vi "Build Action Array.vi"(10 "directions":T2[](array[typedef]), 11 "Action":T1=enum."Move") -> (3 "actions":cluster{"Action":T1, "Direction":T2}[](array[cluster]))   [LabVIEW 2015, in "DS Square.lvlib"]
uses:
  DS Square.lvlib
  Type Defs/Direction Enum.ctl
  Type Defs/SB Type Defs.lvlib
  Type Defs/Action Enum.ctl
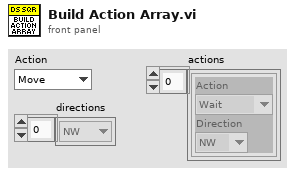
[diagram p1: front panel]
types:
  T1 = typedef "SB Type Defs.lvlib/Action Enum.ctl" = enum16{"Wait", "Move", "Attack", "Replicate"}
  T2 = typedef "SB Type Defs.lvlib/Direction Enum.ctl" = enum16{"NW", "N", "NE", "E", "SE", "S", "SW", "W"}
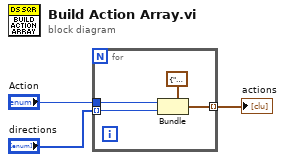
[diagram p0: block diagram]
diagram:
  n1 = for {
    tunnel: "directions" -> [w7] mode=indexing
    tunnel: "Action" -> [w5]
    tunnel: [w4] -> w1 mode=indexing
    n2 = Bundle(cluster=cluster{"Action":T1, "Direction":T2} {"Action"=enum."Wait", "Direction"=enum."NW"}, "Action"=w5, "Direction"=w7) -> (w4:cluster{"Action":T1, "Direction":T2})
  }
  "actions" <- w1
